vi "FTW-JSON-Construct-NewObject.vi"(11 "error in":errorcluster) -> (4 "JSON Object":refnum<data-value>, 15 "error out":errorcluster)   [LabVIEW 2014]
uses:
  core/FTW-JSON-Core-Structure.ctl
panel:
  # "Inputs"
  # "Outputs"
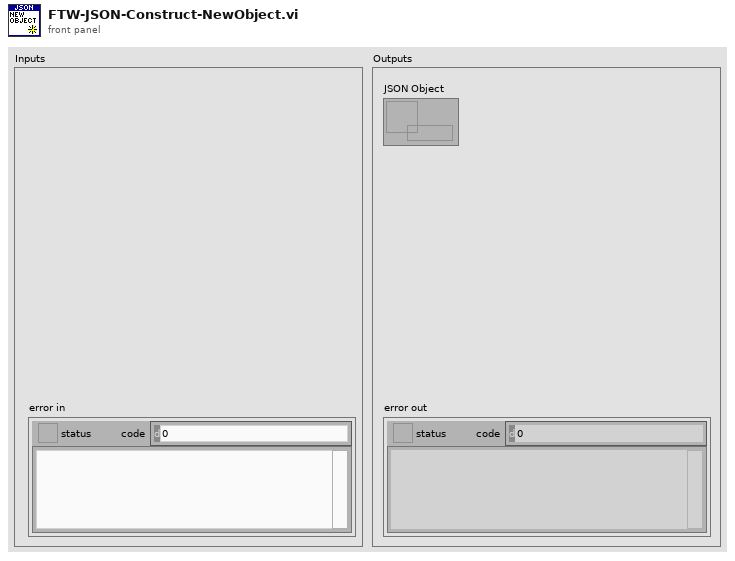
[diagram p1: front panel]
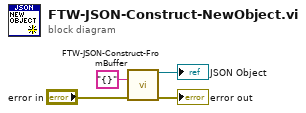
[diagram p0: block diagram]
diagram:
  n1 = call "FTW-JSON-Construct-FromBuffer.vi"("JSON String (UTF-8)"="{}", "error in"="error in") -> ("JSON Object"=→"JSON Object":refnum<data-value>, "error out"=→"error out":errorcluster)  [unwired: 12 in]
